vi "solar_excel Cell Values (Column).vi"(11 "Cells in":string[][](array[string])) -> (3 "Values":string[][](array[string]), 5 "Column Headers":string[](array[string]))   [LabVIEW 2018]
doc: "This removes the Column Headers (first row)."
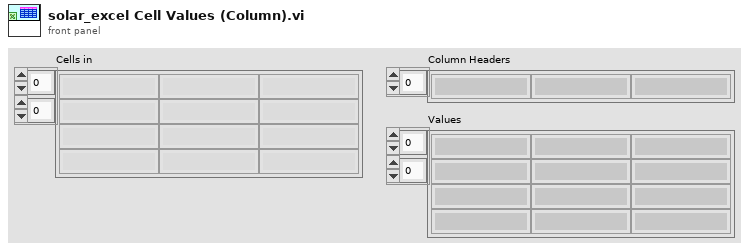
[diagram p1: front panel]
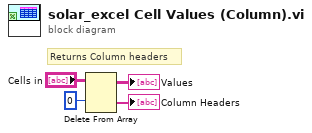
[diagram p0: block diagram]
diagram:
  # "Returns Column headers"
  n1 = Delete From Array(array="Cells in", index (row)=0 ("index")) -> (deleted portion=→"Column Headers":string[], array with subset deleted=→"Values":string[][])  [unwired: 2 in]
